vi "motor_move_piezo.vi"(8 "错误输入（无错误）":errorcluster, 10 "目标位置":dbl, 11 "device index":T1) -> (0 "错误输出":errorcluster, 2 "当前压电位置":dbl, 3 "on target":bool)   [LabVIEW 2017]
uses:
  device index.ctl
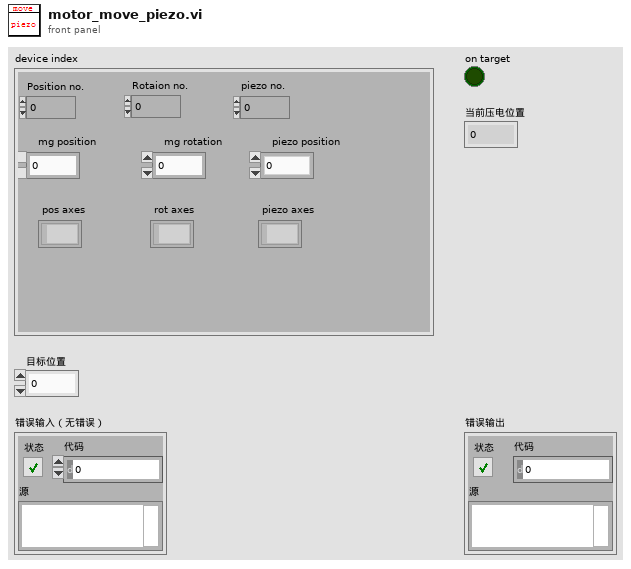
[diagram p1: front panel]
types:
  T1 = typedef "device index.ctl" = cluster{"Position no.":i32, "Rotaion no.":i32, "piezo no.":i32, "mg position":dbl, "mg rotation":dbl, "piezo position":dbl, "pos axes":string[], "rot axes":string[], "piezo axes":string[]}
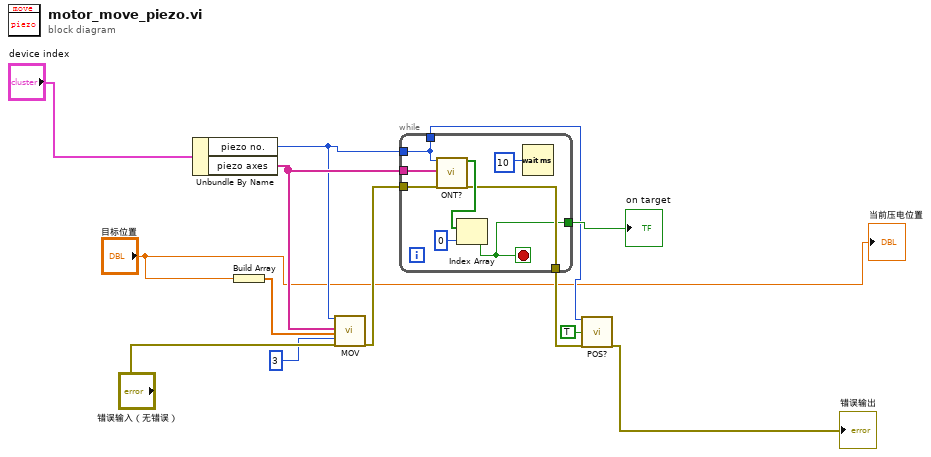
[diagram p0: block diagram]
diagram:
  n1 = Unbundle By Name("device index") -> ("piezo no."=w7:i32, "piezo axes"=w8:string[])
  n2 = Build Array("目标位置") -> (w2:dbl[])
  n3 = call "MOV.vi"("System no."=w7, "Axes to move"=w8, "Position values"=w2, "No.of digits"=i16 3, "error in"="错误输入（无错误）") -> ("error out"=w9:errorcluster)  [unwired: 14 in]
  n4 = while {
    tunnel: w7 -> [w15]
    tunnel: w8 -> [w18]
    tunnel: w9 -> [w17]
    tunnel: [w16] -> w10
    tunnel: [w15] -> w11
    tunnel: [w14] -> w13
    stop <- w14 stop-if-true
    n5 = call "ONT?.vi"("System no."=w15, "Axes to query"=w18, "error in"=w17) -> ("Axis on target?"=w21:bool[], "error out"=w16:errorcluster)  [unwired: 15 in]
    n6 = Index Array(array=w21, index=0 ("索引")) -> (element=w14:bool)
    n7 = Wait (ms)(milliseconds to wait=u32 10 ("等待时间（毫秒）")) -> ()  [unwired: 1 out]
  }
  "on target" <- w13
  n8 = call "POS?.vi"("System no."=w11, "All axes?"=TRUE, "error in"=w10) -> ("error out"=→"错误输出":errorcluster)  [unwired: 15 in, 1 out]
  "当前压电位置" <- "目标位置"
